vi "SPD.Config Read Test02 Strobe_Phase.vi"(8 "Error In":errorcluster, 11 "SPD.Stand Ctrl in":T2 {"spdDeviceSession"."hidSPD.Sturtup Values"."HV_bias" format="%#_6p, V"; "spdDeviceSession"."hidSPD.Sturtup Values"."TSet" format="%#_6p, DegC"; "spdDeviceSession"."hidSPD.Controller"."HV_bias" format="%#_6p, V"; "spdDeviceSession"."hidSPD.Controller"."TSet" format="%#_6p, DegC"}) -> (0 "Error Out":errorcluster, 2 "Stb_Ph Test params":T1, 3 "SPD.Stand Ctrl out":T2 {"spdDeviceSession"."hidSPD.Sturtup Values"."HV_bias" format="%#_6p, V"; "spdDeviceSession"."hidSPD.Sturtup Values"."TSet" format="%#_6p, DegC"; "spdDeviceSession"."hidSPD.Controller"."HV_bias" format="%#_6p, V"; "spdDeviceSession"."hidSPD.Controller"."TSet" format="%#_6p, DegC"})   [LabVIEW 2018]
uses:
  typedefs/SPD.Stand Ctrl.ctl
  Instruments/SPD HID Interface/hidSPDLibForLabView/LibVIs/hidSPD Controls/hidSPD Device Session.ctl
  Instruments/SPD HID Interface/hidSPDLibForLabView/LibVIs/hidSPD Controls/hidSPD Controller.ctl
  Instruments/SPD HID Interface/hidSPDLibForLabView/LibVIs/hidSPD Controls/hidSPD SPD Type.ctl
  Instruments/KC705 DevBoard/typedefs/DevB.Session.ctl
  Instruments/KeySight 53230A/typedefs/FreqC.Session.ctl
  Instruments/KeySight 8164B/KeySight 8164B LAN InstrLib/typedefs/KeySight 8164B control.ctl
  Instruments/LeCroy SDA830/typedefs/LeCroy.Session.ctl
  typedefs/SPD.Events.ctl
  SPD.Config File ctrl.ctl
  <vilib>/Utility/config.llb/Config Data RefNum.ctl
  typedefs/SPD.Meas Result.ctl
  typedefs/SPD.Queues.ctl
  typedefs/SPD.Stand state.ctl
  SPDTests/SubTests/02_Strobe_Phase Test/SPD.Strobe_Phase Test Params.ctl
  <vilib>/Utility/config.llb/Read Key (I32).vi
  <vilib>/Utility/config.llb/Read Key (Double).vi
  <vilib>/Utility/config.llb/NI_LVConfig.lvlib
  Instruments/KeySight 8164B/KeySight 8164B LAN InstrLib.lvlib
  Instruments/SPD HID Interface/hidSPDLibForLabView/hidSPDLibForLabView.lvlib
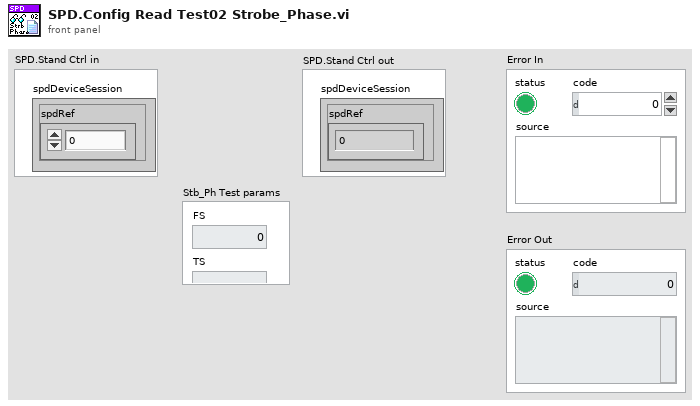
[diagram p1: front panel]
types:
  T1 = typedef "SPD.Strobe_Phase Test Params.ctl" = cluster{"FS":i32, "TS":i32, "Wavelength":dbl, "Punits":i32, "Pset":dbl, "Att":dbl, "ph_quick_start":i32, "ph_quick_stop":i32, "ph_quick_step":i32, "gate_quick":dbl, "ph_precise_step":i32, "gate_precise":dbl}
  T2 = typedef "SPD.Stand Ctrl.ctl" = cluster{"spdDeviceSession":T3, "DevBSession":T6, "FreqCSession":T7, "8164BSession":T8, "LeCroySession":T9, "Events":T10, "configFile":T11, "SPD.Result":T13, "SPD.Queues":T14, "Console":refnum<vi>}
  T3 = typedef "hidSPDLibForLabView.lvlib/hidSPD Device Session.ctl" = cluster{"spdRef":u64, "connected":bool, "spdName":string, "hidSPD.Controller":T4, "hidSPD.Sturtup Values":T4, "SPD Type":T5}
  T4 = typedef "hidSPDLibForLabView.lvlib/hidSPD Controller.ctl" = cluster{"TSet":sgl, "HV_bias":sgl, "DDS_stb_code":u16}
  T5 = typedef "hidSPDLibForLabView.lvlib/hidSPD SPD Type.ctl" = enum16{"Free Run", "Gate"}
  T6 = typedef "DevB.Session.ctl" = cluster{"DevBRef":refnum<visa-resource-name>, "connected":bool}
  T7 = typedef "FreqC.Session.ctl" = cluster{"FreqCRef":refnum<visa-resource-name>, "timeout":dbl, "Gate":dbl, "connected":bool}
  T8 = typedef "KeySight 8164B LAN InstrLib.lvlib/KeySight 8164B control.ctl" = cluster{"Connection ID":refnum<k5>, "Connected":bool, "Info":string, "Slots Info":string[]}
  T9 = typedef "LeCroy.Session.ctl" = cluster{"LeCroySession":refnum<visa-resource-name>, "connected":bool}
  T10 = typedef "SPD.Events.ctl" = cluster{"DCRTest":refnum<user-event>, "Stop":refnum<user-event>}
  T11 = typedef "SPD.Config File ctrl.ctl" = cluster{"configFile ref":T12, "configFile path":path, "equipmentFile ref":T12}
  T12 = typedef "NI_LVConfig.lvlib/Config Data RefNum.ctl" = refnum<k1>
  T13 = typedef "SPD.Meas Result.ctl" = cluster{"HV_Bias":dbl[][][], "Stb_code":dbl[], "Temprature":dbl[], "Data":dbl[][][][], "DateTime":string}
  T14 = typedef "SPD.Queues.ctl" = cluster{"state queue":refnum<queue>}
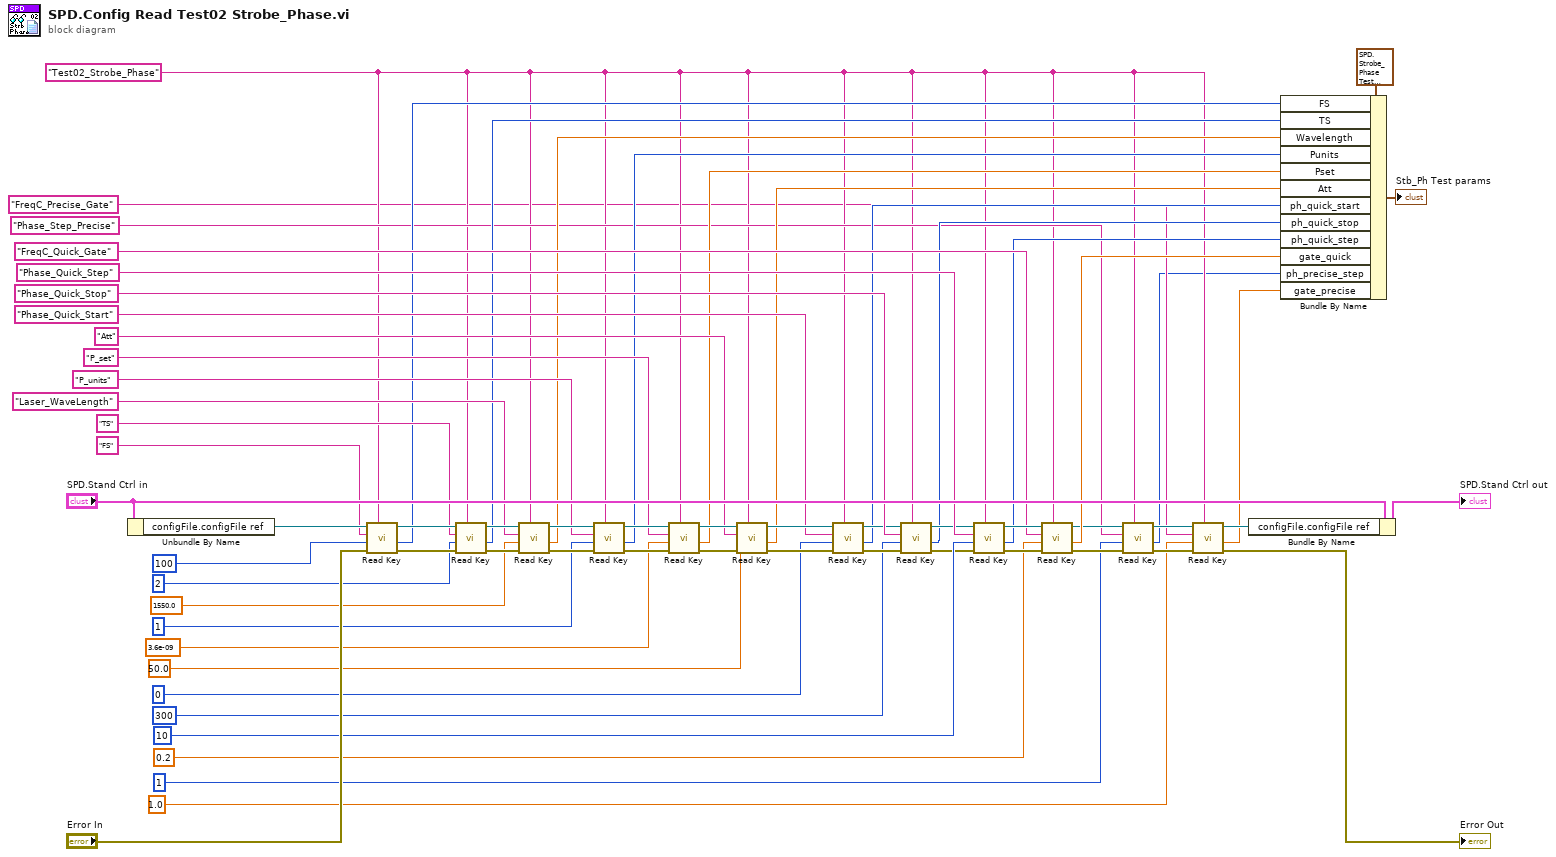
[diagram p0: block diagram]
diagram:
  w11 = "Test02_Strobe_Phase" ("section")
  n1 = Unbundle By Name("SPD.Stand Ctrl in") -> ("configFile.configFile ref"=w65:T12)
  n2 = call-poly <vilib>:"Read Key.vi"("section"=w11, "error in (no error)"="Error In", "default value"=100, "key"="FS", "refnum"=w65) -> ("error out"=w61:errorcluster, "value"=w25:i32, "refnum out"=w60:T12)  [unwired: 3 in, 1 out]
  n3 = call-poly <vilib>:"Read Key.vi"("section"=w11, "error in (no error)"=w61, "default value"=2, "key"="TS", "refnum"=w60) -> ("error out"=w56:errorcluster, "value"=w24:i32, "refnum out"=w57:T12)  [unwired: 3 in, 1 out]
  n4 = call-poly <vilib>:"Read Key.vi"("section"=w11, "error in (no error)"=w56, "default value"=1550.0, "key"="Laser_WaveLength", "refnum"=w57) -> ("error out"=w52:errorcluster, "value"=w23:dbl, "refnum out"=w53:T12)  [unwired: 3 in, 1 out]
  n5 = call-poly <vilib>:"Read Key.vi"("section"=w11, "error in (no error)"=w52, "default value"=1, "key"="P_units", "refnum"=w53) -> ("error out"=w48:errorcluster, "value"=w22:i32, "refnum out"=w49:T12)  [unwired: 3 in, 1 out]
  n6 = call-poly <vilib>:"Read Key.vi"("section"=w11, "error in (no error)"=w48, "default value"=3.6e-09, "key"="P_set", "refnum"=w49) -> ("error out"=w42:errorcluster, "value"=w21:dbl, "refnum out"=w45:T12)  [unwired: 3 in, 1 out]
  n7 = call-poly <vilib>:"Read Key.vi"("section"=w11, "error in (no error)"=w42, "default value"=50.0, "key"="Att", "refnum"=w45) -> ("error out"=w33:errorcluster, "value"=w20:dbl, "refnum out"=w34:T12)  [unwired: 3 in, 1 out]
  n8 = call-poly <vilib>:"Read Key.vi"("section"=w11, "error in (no error)"=w33, "default value"=0, "key"="Phase_Quick_Start", "refnum"=w34) -> ("error out"=w35:errorcluster, "value"=w19:i32, "refnum out"=w28:T12)  [unwired: 3 in, 1 out]
  n9 = call-poly <vilib>:"Read Key.vi"("section"=w11, "error in (no error)"=w35, "default value"=300, "key"="Phase_Quick_Stop", "refnum"=w28) -> ("error out"=w26:errorcluster, "value"=w18:i32, "refnum out"=w27:T12)  [unwired: 3 in, 1 out]
  n10 = call-poly <vilib>:"Read Key.vi"("section"=w11, "error in (no error)"=w26, "default value"=10, "key"="Phase_Quick_Step", "refnum"=w27) -> ("error out"=w40:errorcluster, "value"=w17:i32, "refnum out"=w41:T12)  [unwired: 3 in, 1 out]
  n11 = call-poly <vilib>:"Read Key.vi"("section"=w11, "error in (no error)"=w40, "default value"=0.2, "key"="FreqC_Quick_Gate", "refnum"=w41) -> ("error out"=w14:errorcluster, "value"=w16:dbl, "refnum out"=w15:T12)  [unwired: 3 in, 1 out]
  n12 = call-poly <vilib>:"Read Key.vi"("section"=w11, "error in (no error)"=w14, "default value"=1, "key"="Phase_Step_Precise", "refnum"=w15) -> ("error out"=w10:errorcluster, "value"=w3:i32, "refnum out"=w12:T12)  [unwired: 3 in, 1 out]
  n13 = call-poly <vilib>:"Read Key.vi"("section"=w11, "error in (no error)"=w10, "default value"=1.0, "key"="FreqC_Precise_Gate", "refnum"=w12) -> ("error out"=→"Error Out":errorcluster, "value"=w2:dbl, "refnum out"=w8:T12)  [unwired: 3 in, 1 out]
  n14 = Bundle By Name(cluster="SPD.Stand Ctrl in", "configFile.configFile ref"=w8) -> (→"SPD.Stand Ctrl out":T2)
  n15 = Bundle By Name(cluster=T1 {"FS"=0, "TS"=0, "Wavelength"=0.0, "Punits"=0, "Pset"=0.0, "Att"=0.0, "ph_quick_start"=0, "ph_quick_stop"=0, "ph_quick_step"=0, "gate_quick"=0.0, "ph_precise_step"=0, "gate_precise"=0.0} ("SPD.Strobe_Phase Test Params"), "FS"=w25, "TS"=w24, "Wavelength"=w23, "Punits"=w22, "Pset"=w21, "Att"=w20, "ph_quick_start"=w19, "ph_quick_stop"=w18, "ph_quick_step"=w17, "gate_quick"=w16, "ph_precise_step"=w3, "gate_precise"=w2) -> (→"Stb_Ph Test params":T1)
